vi "ArduinoConfig.vi"(2 "error in (no error)":errorcluster) -> (0 "error out":errorcluster, 1 "VISA resource name":refnum<visa-resource-name>)   [LabVIEW 2013]
uses:
  global/InstrumentSetup.vi
panel:
  in  "T sensor":enum16{"SHT", "DS"}(ring)
  in  "Blank Button":bool
  out "Programm uploaded?":string
  in  "OK Button":bool
  in  "VISA resource name":refnum<visa-resource-name>="COM4"
  # "Arduino Uno Edgesense"
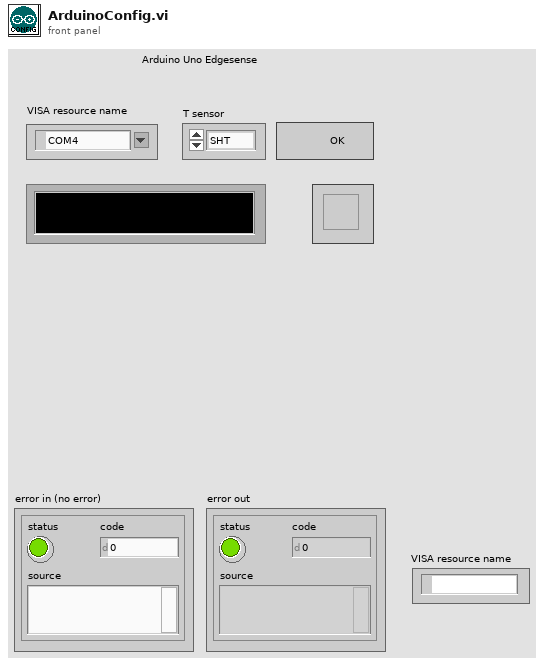
[diagram p1: front panel]
types:
  T1 = cluster{"Readout":enum16{"Arduino Uno", "Nothing"}, "VISA address":refnum<visa-resource-name>, "VISA address LED array":refnum<visa-resource-name>, "T sensor":enum16{"SHT", "DS"}}
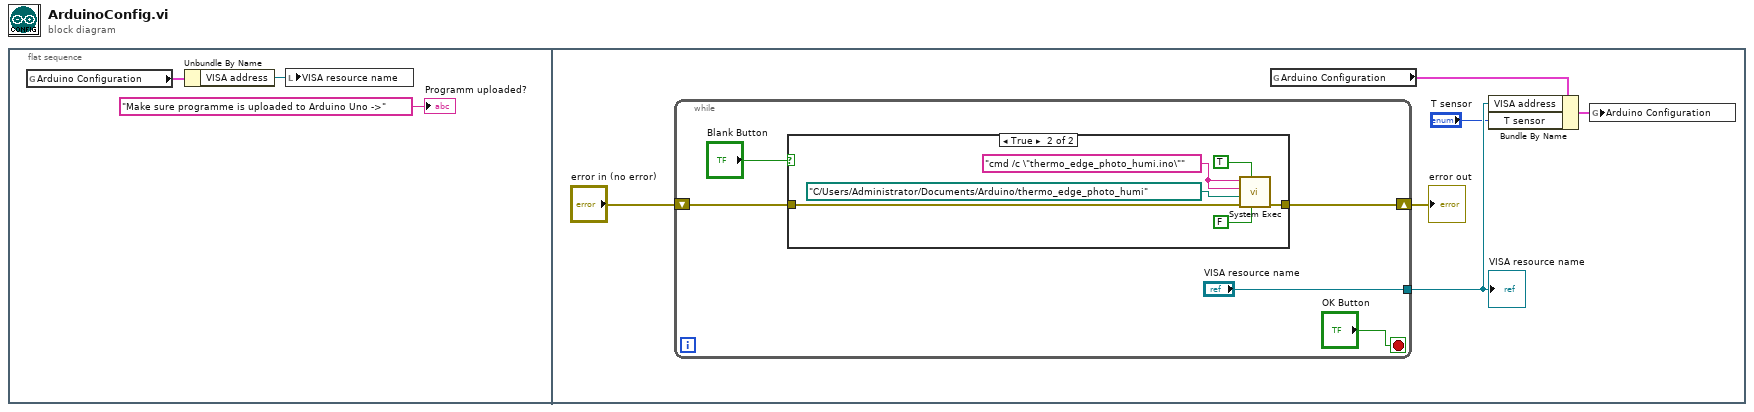
[diagram p0: block diagram]
diagram:
  n1 = flat-sequence {
    frame #0 {
      n2 = global read "InstrumentSetup.vi" "Arduino Configuration"() -> (w2:T1)
      n3 = Unbundle By Name(w2) -> ("VISA address"=w1:refnum<visa-resource-name>)
      n4 = local write "VISA resource name"(w1) -> ()
      "Programm uploaded?" <- "Make sure programme is uploaded to Arduino Uno ->"
    }
    frame #1 {
      n5 = while {
        tunnel: ["VISA resource name"] -> w6
        shift-right: [w10] -> w8
        shift-left: "error in (no error)" -> [w11]
        stop <- "OK Button" stop-if-true
        n6 = case shown="True" "Blank Button" {
          tunnel: w11 -> [w15 w21]
          tunnel: [w15 w20] -> w10
          frame False {
          }
          frame True {
            w17 = "cmd /c \"thermo_edge_photo_humi.ino\""
            n7 = call <vilib>:"System Exec.vi"("run minimized? (F)"=FALSE, "wait until completion? (T)"=TRUE, "error in (no error)"=w21, "working directory"=path "C:/Users/Administrator/Documents/Arduino/thermo_edge_photo_humi", "standard input"=w17, "command line"=w17) -> ("error out"=w20:errorcluster)  [unwired: 2 in, 3 out]
          }
        }
      }
      "error out" <- w8
      "VISA resource name" <- w6
      n8 = global read "InstrumentSetup.vi" "Arduino Configuration"() -> (w7:T1)
      n9 = Bundle By Name(cluster=w7, "VISA address"=w6, "T sensor"="T sensor") -> (w4:T1)
      n10 = global write "InstrumentSetup.vi" "Arduino Configuration"(w4) -> ()
    }
  }
